vi "Get Channel.vi"(8 "error in (no error)":errorcluster, 10 "channel":T2=1 min=1 max=8 step=1, 11 "VISA Refnum in":refnum<visa-resource-name>="COM1") -> (0 "error out":errorcluster, 2 "channelProperties":T1={"channel"=1, "gain"=enum."10", "input"=enum."SE+", "shunt"=enum."50", "couple"=enum."DC", "filter"=enum."ON"} {"channel" min=1 max=8 step=1}, 3 "VISA Refnum out":refnum<visa-resource-name>)   [LabVIEW 2019, in "KH7008.lvlib"]
uses:
  KH7008.lvlib
  typedefs/channel--numeric.ctl
  typedefs/channelProperties--Cluster.ctl
  typedefs/gain--enum.ctl
  typedefs/Input--Enum.ctl
  typedefs/shunt--enum.ctl
  typedefs/couple--Enum.ctl
  typedefs/Filter--Enum.ctl
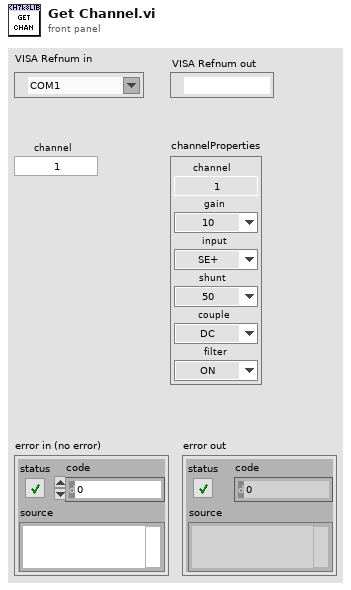
[diagram p1: front panel]
types:
  T1 = typedef "KH7008.lvlib/channelProperties--Cluster.ctl" = cluster{"channel":T2, "gain":T3, "input":T4, "shunt":T5, "couple":T6, "filter":T7}
  T2 = typedef "KH7008.lvlib/channel--numeric.ctl" = u16
  T3 = typedef "KH7008.lvlib/gain--enum.ctl" = enum16{"1", "10", "100", "1000"}
  T4 = typedef "KH7008.lvlib/input--enum.ctl" = enum16{"OFF", "SE+", "SE-", "DIFF"}
  T5 = typedef "KH7008.lvlib/shunt--enum.ctl" = enum16{"Open", "50", "500", "5k", "50k", "10M"}
  T6 = typedef "KH7008.lvlib/couple--enum.ctl" = enum16{"AC", "DC"}
  T7 = typedef "KH7008.lvlib/filter--enum.ctl" = enum16{"OFF", "ON"}
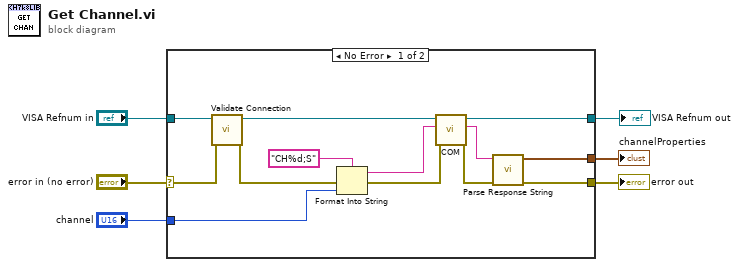
[diagram p0: block diagram]
diagram:
  n1 = case shown="No Error" "error in (no error)" {
    selector: "error in (no error)" -> [w8 w21]
    tunnel: [w19 w21] -> w6
    tunnel: [w17 _] -> w5
    tunnel: "channel" -> [w16 _]
    tunnel: [w18 w20] -> w2
    tunnel: "VISA Refnum in" -> [w9 w20]
    frame No Error {
      n2 = call "Validate Connection.vi"("error in (no error)"=w8, "VISA Refnum in"=w9) -> ("error out"=w7:errorcluster, "VISA Refnum out"=w10:refnum<visa-resource-name>)  [unwired: 8 in]
      n3 = Format Into String(format string="CH%d;S", error in=w7, w16) -> (resulting string=w12:string, error out=w13:errorcluster)  [unwired: 1 in]
      n4 = call "COM.vi"("error in (no error)"=w13, "Command"=w12, "VISA Refnum in"=w10) -> ("error out"=w15:errorcluster, "Response"=w14:string, "VISA Refnum out"=w18:refnum<visa-resource-name>)  [unwired: 6 in]
      n5 = call "Parse Response String.vi"("error in (no error)"=w15, "Response String"=w14) -> ("error out"=w19:errorcluster, "channelProperties"=w17:T1)  [unwired: 8 in]
    }
    frame Error {
    }
  }
  "error out" <- w6
  "VISA Refnum out" <- w2
  "channelProperties" <- w5
